vi "Set Transfer Group Timing.vi"(7 "priority (100)":u64=100, 8 "error in (no error)":errorcluster, 9 "offset (0)":u64, 10 "decimation (1)":u64=1, 11 "transfer group in":T1={"name"="Group", "direction"=enum."Tx", "cycle timing"={"priority"=100, "decimation"=1, "offset"=0}, "thread index"=255, "settings"=[], "transfers"=[], "timeout behavior"=enum."Increment Late Count", "convert buffers"=FALSE} {"transfers"."channels"."string offset" format="%d bytes"}) -> (0 "error out":errorcluster, 3 "transfer group out":T1={"name"="Group", "direction"=enum."Tx", "cycle timing"={"priority"=100, "decimation"=1, "offset"=0}, "thread index"=255, "settings"=[], "transfers"=[], "timeout behavior"=enum."Increment Late Count", "convert buffers"=FALSE} {"transfers"."channels"."string offset" format="%d bytes"})   [LabVIEW 2017, in "DSF Core.lvlib" / "Configuration Session.lvclass"]
uses:
  Configuration Session.lvclass
  Typedefs/DSF Engine Transfer Group Configuration.ctl
  Typedefs/DSF Direction.ctl
  Typedefs/DSF Timing Info.ctl
  Typedefs/DSF Settings Info.ctl
  Typedefs/DSF Engine Transfer Configuration.ctl
  Typedefs/DSF Byte Order.ctl
  Typedefs/DSF Engine Channel Configuration.ctl
  Typedefs/DSF Data Type.ctl
  Typedefs/DSF Timeout Behavior.ctl
  DSF Core.lvlib
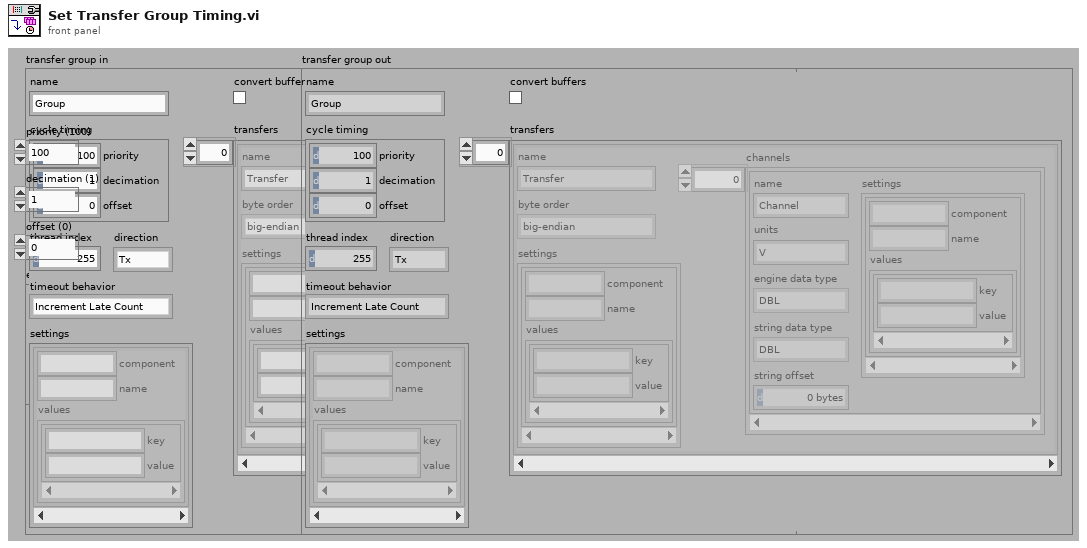
[diagram p1: front panel]
types:
  T1 = typedef "DSF Core.lvlib/DSF Engine Transfer Group Configuration.ctl" = cluster{"name":string, "direction":T2, "cycle timing":T3, "thread index":u8, "settings":T4, "transfers":T5[], "timeout behavior":T9, "convert buffers":bool}
  T2 = typedef "DSF Core.lvlib/DSF Direction.ctl" = enum8{"Tx", "Rx"}
  T3 = typedef "DSF Core.lvlib/DSF Timing Info.ctl" = cluster{"priority":u64, "decimation":u64, "offset":u64}
  T4 = typedef "DSF Core.lvlib/DSF Settings Info.ctl" = cluster{"component":string, "name":string, "values":cluster{"key":string, "value":string}[]}[]
  T5 = typedef "DSF Core.lvlib/DSF Engine Transfer Configuration.ctl" = cluster{"name":string, "byte order":T6, "settings":T4, "channels":T7[]}
  T6 = typedef "DSF Core.lvlib/DSF Byte Order.ctl" = enum8{"big-endian", "little-endian"}
  T7 = typedef "DSF Core.lvlib/DSF Engine Channel Configuration.ctl" = cluster{"string offset":u64, "name":string, "units":string, "engine data type":T8, "string data type":T8, "settings":T4}
  T8 = typedef "DSF Core.lvlib/DSF Data Type.ctl" = enum8{"Bool", "SGL", "DBL", "I8", "I16", "I32", "I64", "U8", "U16", "U32", "U64"}
  T9 = typedef "DSF Core.lvlib/DSF Timeout Behavior.ctl" = enum8{"Increment Late Count", "Throw Error"}
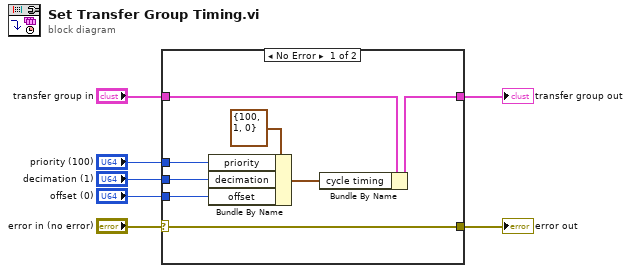
[diagram p0: block diagram]
diagram:
  n1 = case shown="No Error" "error in (no error)" {
    selector: "error in (no error)" -> [w13 w17]
    tunnel: [w13 w17] -> w7
    tunnel: [w14 w16] -> w4
    tunnel: "transfer group in" -> [w15 w16]
    tunnel: "offset (0)" -> [w11 _]
    tunnel: "decimation (1)" -> [w10 _]
    tunnel: "priority (100)" -> [w9 _]
    frame No Error {
      n2 = Bundle By Name(cluster=T3 {"priority"=100, "decimation"=1, "offset"=0} ("cycle timing"), "priority"=w9, "decimation"=w10, "offset"=w11) -> (w8:T3)
      n3 = Bundle By Name(cluster=w15, "cycle timing"=w8) -> (w14:T1)
    }
    frame Error {
    }
  }
  "error out" <- w7
  "transfer group out" <- w4
